vi "Event Is Nested.vi"(10 "Alias":string, 11 "Base Queue Actor in":refnum<class "Base Queue Actor.lvclass">) -> (2 "Event Is Nested?":bool)   [LabVIEW 2021, in "jettl.lvlib" / "Base Queue Actor.lvclass"]
uses:
  Base Queue Actor.lvclass
  Base Queue Actor.lvclass/Base Queue Actor.ctl
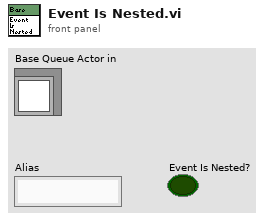
[diagram p1: front panel]
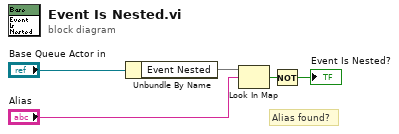
[diagram p0: block diagram]
diagram:
  # "Alias found?"
  n1 = Unbundle By Name("Base Queue Actor in") -> ("Event Nested"=w5:map{string, refnum<data-value>})
  n2 = Look In Map(map=w5, key="Alias") -> (key not found?=w4:bool)  [unwired: 1 in, 1 out]
  n3 = Not(x=w4) -> (.not. x?=→"Event Is Nested?":bool)
